vi "CompStopTrig.vi"(0 "reference":refnum<k24>, 5 "error in (no error)":errorcluster) -> (8 "DigitalPatternTriggerSense":i32(ring) items=["AbovePattern", "BelowPattern", "EqualPattern", "NotEqualPattern"], 10 "TriggerChannelStr":string, 11 "TriggerChannel":i32, 12 "Type":i32(ring) items=["None", "AnalogSW", "DigitalPattern", "Counter"], 13 "AnalogSWTriggerSense":i32(ring) items=["AboveLevel", "BelowLevel", "EqualLevel", "NotEqualLevel", "RisingEdge", "FallingEdge"], 14 "reference out":refnum<k24>, 16 "CounterChannelTriggerSense":i32(ring) items=["AboveCount", "BelowCount", "EqualCount", "NotEqualCount", "RisingCount", "FallingCount"], 17 "Level":dbl, 18 "Variance":dbl, 19 "error out":errorcluster)   [LabVIEW 2009]
uses:
  C:/Program Files/National Instruments/LabVIEW 2009/vi.lib/ULx/ULx_LV.dll
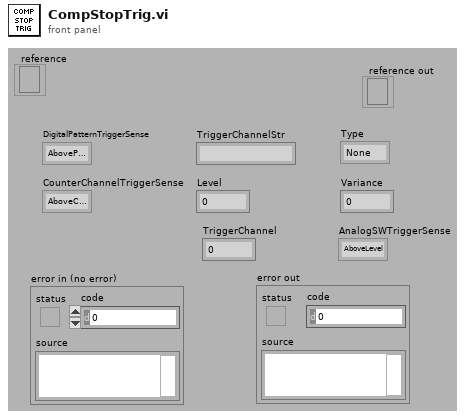
[diagram p1: front panel]
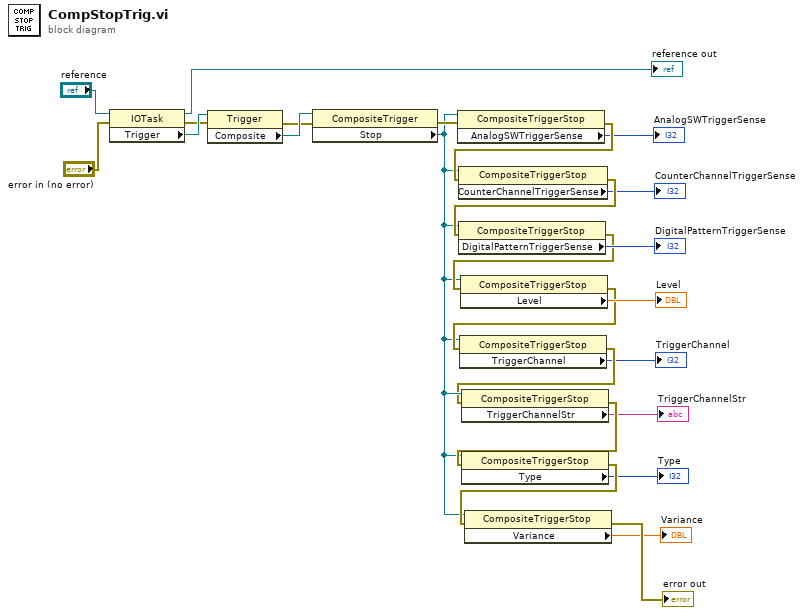
[diagram p0: block diagram]
diagram:
  n1 = property class="IOTask"(reference="reference", error in="error in (no error)") -> (reference out=→"reference out":refnum<k24>, error out=w20:errorcluster, "Trigger"=w25:refnum<k24>)
  n2 = property class="Trigger"(reference=w25, error in=w20) -> (error out=w19:errorcluster, "Composite"=w24:refnum<k24>)  [unwired: 1 out]
  n3 = property class="CompositeTrigger"(reference=w24, error in=w19) -> (error out=w18:errorcluster, "Stop"=w3:refnum<k24>)  [unwired: 1 out]
  n4 = property class="CompositeTriggerStop"(reference=w3, error in=w18) -> (error out=w17:errorcluster, "AnalogSWTriggerSense"=→"AnalogSWTriggerSense":i32)  [unwired: 1 out]
  n5 = property class="CompositeTriggerStop"(reference=w3, error in=w17) -> (error out=w16:errorcluster, "CounterChannelTriggerSense"=→"CounterChannelTriggerSense":i32)  [unwired: 1 out]
  n6 = property class="CompositeTriggerStop"(reference=w3, error in=w16) -> (error out=w6:errorcluster, "DigitalPatternTriggerSense"=→"DigitalPatternTriggerSense":i32)  [unwired: 1 out]
  n7 = property class="CompositeTriggerStop"(reference=w3, error in=w6) -> (error out=w4:errorcluster, "Level"=→"Level":dbl)  [unwired: 1 out]
  n8 = property class="CompositeTriggerStop"(reference=w3, error in=w4) -> (error out=w2:errorcluster, "TriggerChannel"=→"TriggerChannel":i32)  [unwired: 1 out]
  n9 = property class="CompositeTriggerStop"(reference=w3, error in=w2) -> (error out=w15:errorcluster, "TriggerChannelStr"=→"TriggerChannelStr":string)  [unwired: 1 out]
  n10 = property class="CompositeTriggerStop"(reference=w3, error in=w15) -> (error out=w14:errorcluster, "Type"=→"Type":i32)  [unwired: 1 out]
  n11 = property class="CompositeTriggerStop"(reference=w3, error in=w14) -> (error out=→"error out":errorcluster, "Variance"=→"Variance":dbl)  [unwired: 1 out]
